vi "init.vi"(8 "error in (no error)":errorcluster, 11 "Fake ILC in":refnum<class "Fake ILC.lvclass">) -> (0 "error out":errorcluster, 3 "Fake ILC out":refnum<class "Fake ILC.lvclass">)   [LabVIEW 2015, in "Fake ILC.lvclass"]
uses:
  Fake ILC.lvclass
  Fake ILC.lvclass/Fake ILC.ctl
  <userlib>/Common/ILC/ILC/ILC.lvclass
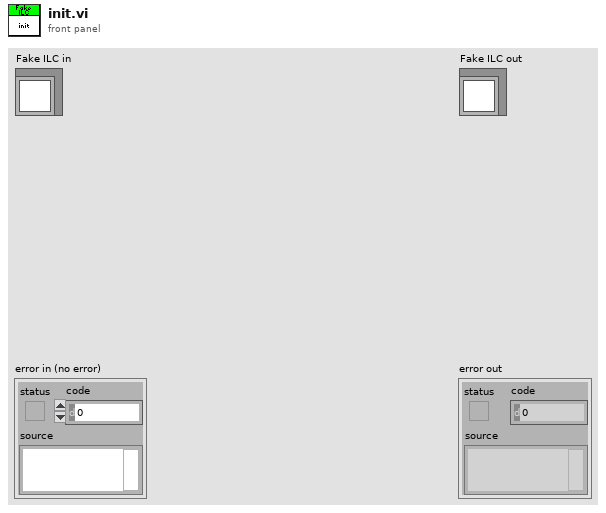
[diagram p1: front panel]
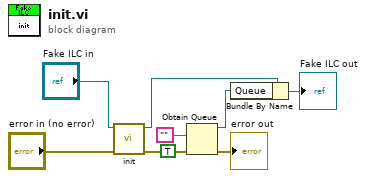
[diagram p0: block diagram]
diagram:
  n1 = call-parent "init.vi"("error in (no error)"="error in (no error)", "ILC in"="Fake ILC in") -> ("error out"=w4:errorcluster, "ILC out"=w7:refnum<class "Fake ILC.lvclass">)  [unwired: 8 in]
  n2 = Obtain Queue(element data type="", create if not found? (T)=TRUE, error in (no error)=w4) -> (queue out=w2:refnum<queue>, error out=→"error out":errorcluster)  [unwired: 2 in, 1 out]
  n3 = Bundle By Name(cluster=w7, "Queue"=w2) -> (→"Fake ILC out":refnum<class "Fake ILC.lvclass">)
